vi "Array Max & Min Numeric.vi"(7 "JSON Array":refnum<class "JSON Helper.lvclass">, 11 "error in (no error)":errorcluster) -> (4 "max value":refnum<class "JSON Numeric.lvclass">, 6 "max index":i32, 8 "min value":refnum<class "JSON Numeric.lvclass">, 10 "min index":i32, 15 "error out":errorcluster)   [LabVIEW 2016]
uses:
  JSON Helper/JSON Helper.lvclass
  JSON Helper/To More Specific Type (Numeric).vi
  JSON Numeric/JSON Numeric.lvclass
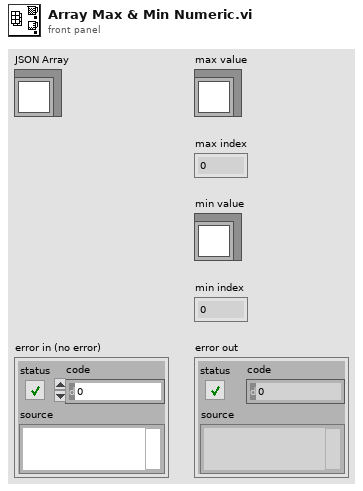
[diagram p1: front panel]
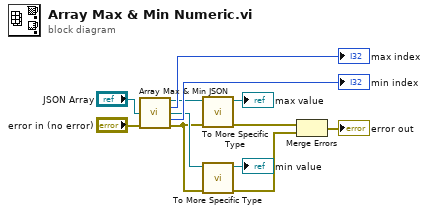
[diagram p0: block diagram]
diagram:
  n1 = call "Array Max & Min JSON.vi"("JSON Array"="JSON Array", "error in (no error)"="error in (no error)") -> ("max value"=w8:refnum<class "JSON Null.lvclass">, "max index"=→"max index":i32, "min value"=w7:refnum<class "JSON Null.lvclass">, "min index"=→"min index":i32, "error out"=w6:errorcluster)  [unwired: 9 in]
  n2 = call-poly "To More Specific Type.vi"("error in (no error)"=w6, "JSON Datatype in"=w8) -> ("error out"=w3:errorcluster, "JSON Numeric out"=→"max value":refnum<class "JSON Numeric.lvclass">)  [unwired: 8 in]
  n3 = call-poly "To More Specific Type.vi"("error in (no error)"=w6, "JSON Datatype in"=w7) -> ("error out"=w5:errorcluster, "JSON Numeric out"=→"min value":refnum<class "JSON Numeric.lvclass">)  [unwired: 8 in]
  n4 = Merge Errors(w3, w5) -> (→"error out":errorcluster)
